vi "Acquire Lock.vi"(7 "Lock Type":T1, 8 "error in (no error)":errorcluster, 9 "Timeout ms":i32, 11 "WebSocket Client in":refnum<class "WebSocket Client.lvclass">) -> (0 "error out":errorcluster, 1 "Remaining  Timeout":i32, 2 "Acquired":bool, 3 "WebSocket Client out":refnum<class "WebSocket Client.lvclass">)   [LabVIEW 2020, in "HTTP Server.lvlib" / "WebSocket Client.lvclass"]
uses:
  WebSocket Client.lvclass
  Lock Type.ctl
  WebSocket Client.lvclass/WebSocket Client.ctl
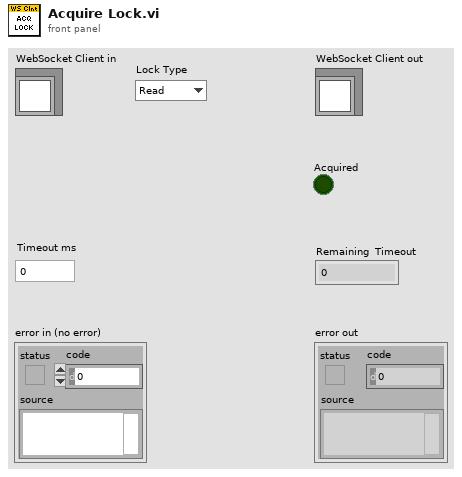
[diagram p1: front panel]
types:
  T1 = typedef "HTTP Server.lvlib/WebSocket Client.lvclass/Lock Type.ctl" = enum16{"Read", "Write"}
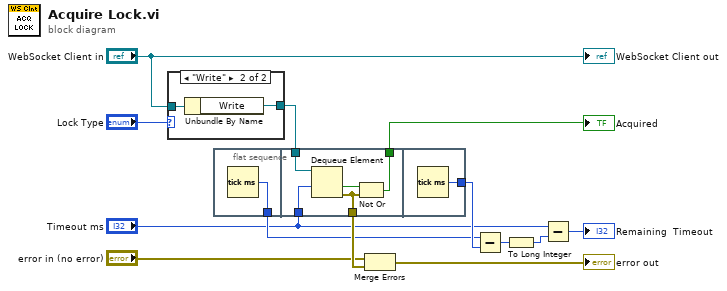
[diagram p0: block diagram]
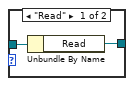
[diagram p2: hidden frame]
diagram:
  n1 = case shown="\"Write\"" "Lock Type" {
    tunnel: "WebSocket Client in" -> [w15 w17]
    tunnel: [w14 w16] -> w13
    frame "Read" {
      n2 = Unbundle By Name(w15) -> ("Read"=w14:refnum<queue>)
    }
    frame "Write" {
      n3 = Unbundle By Name(w17) -> ("Write"=w16:refnum<queue>)
    }
  }
  n4 = flat-sequence {
    tunnel: [w18] -> w10
    tunnel: w13 -> [w23]
    tunnel: [w20] -> w12
    tunnel: [w19] -> w1
    tunnel: "Timeout ms" -> [w22]
    tunnel: [w24] -> w11
    frame #0 {
      n5 = Tick Count (ms)() -> (millisecond timer value=w18:u32)
    }
    frame #1 {
      n6 = Dequeue Element(queue=w23, timeout in ms (-1)=w22) -> (timed out?=w21:bool, error out=w20:errorcluster)  [unwired: 1 in, 2 out]
      n7 = Not Or(1:w20, 2:w21) -> (0:w19:bool)
    }
    frame #2 {
      n8 = Tick Count (ms)() -> (millisecond timer value=w24:u32)
    }
  }
  n9 = Merge Errors("error in (no error)", w12) -> (→"error out":errorcluster)
  n10 = Subtract(x=w10, y=w11) -> (x-y=w9:u32)
  n11 = To Long Integer(number=w9) -> (32bit integer=w8:i32)
  n12 = Subtract(x="Timeout ms", y=w8) -> (x-y=→"Remaining  Timeout":i32)
  "WebSocket Client out" <- "WebSocket Client in"
  "Acquired" <- w1
